vi "Chroma 1905x Series Source Mode Query.vi"(8 "error in (no error)":errorcluster, 11 "VISA resource name":refnum<visa-resource-name>) -> (0 "error out":errorcluster, 2 "Mode":string, 3 "VISA resource name out":refnum<visa-resource-name>)   [LabVIEW 2025]
doc: "Chroma\n5 Clock Tower Place Suite 210\nMaynard, MA 01754\nTel: 1 800 253-1230\nTel: 1 877 4 A HIPOT\nFax: 1 978-461-4295\nWebsite: www.chroma.com"
panel:
  in  "Step":u32=1 min=1 max=99 step=1
  # "MODE by Step query"
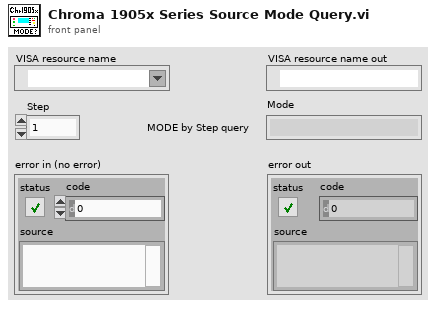
[diagram p1: front panel]
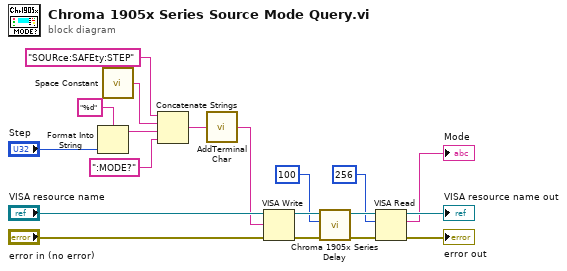
[diagram p0: block diagram]
diagram:
  n1 = Format Into String(format string="%d", "Step") -> (resulting string=w5:string)  [unwired: 2 in, 1 out]
  n2 = call <vilib>:"Space Constant.vi"() -> ("String"=w3:string)
  n3 = Concatenate Strings("SOURce:SAFEty:STEP", w3, w5, ":MODE?") -> (w1:string)
  n4 = call "AddTerminal Char.vi"("Cmd string"=w1) -> ("Concatenated String"=w11:string)  [unwired: 4 in]
  n5 = VISA Write(VISA resource name="VISA resource name", write buffer=w11, error in (no error)="error in (no error)") -> (VISA resource name out=w17:refnum<visa-resource-name>, error out=w19:errorcluster)  [unwired: 1 out]
  n6 = call "Chroma 1905x Series Delay.vi"("error in (no error)"=w19, "Time Delay [ms]"=u32 100 ("Time Delay ms"), "VISA resource name"=w17) -> ("error out"=w18:errorcluster, "VISA resource name 2"=w16:refnum<visa-resource-name>)  [unwired: 7 in]
  n7 = VISA Read(VISA resource name=w16, byte count=u32 256, error in (no error)=w18) -> (VISA resource name out=→"VISA resource name out":refnum<visa-resource-name>, read buffer=→"Mode":string, error out=→"error out":errorcluster)  [unwired: 1 out]
